vi "Part 2.vi"(11 "Input":string) -> (3 "Output":i64)   [LabVIEW 2021]
uses:
  b049b533-3b1e-4f4f-af40-132109b76cf6.vi
  <userlib>/_OpenG.lib/string/string.llb/Convert EOLs (String)__ogtk.vi
panel:
  in  "Numeric":i32=20
  out "Rocks":i32
  out "XY Graph":cluster{i32[], i32[]}[](graph)
  out "Time":dbl
  out "Pass?":bool
  in  "Test":i32
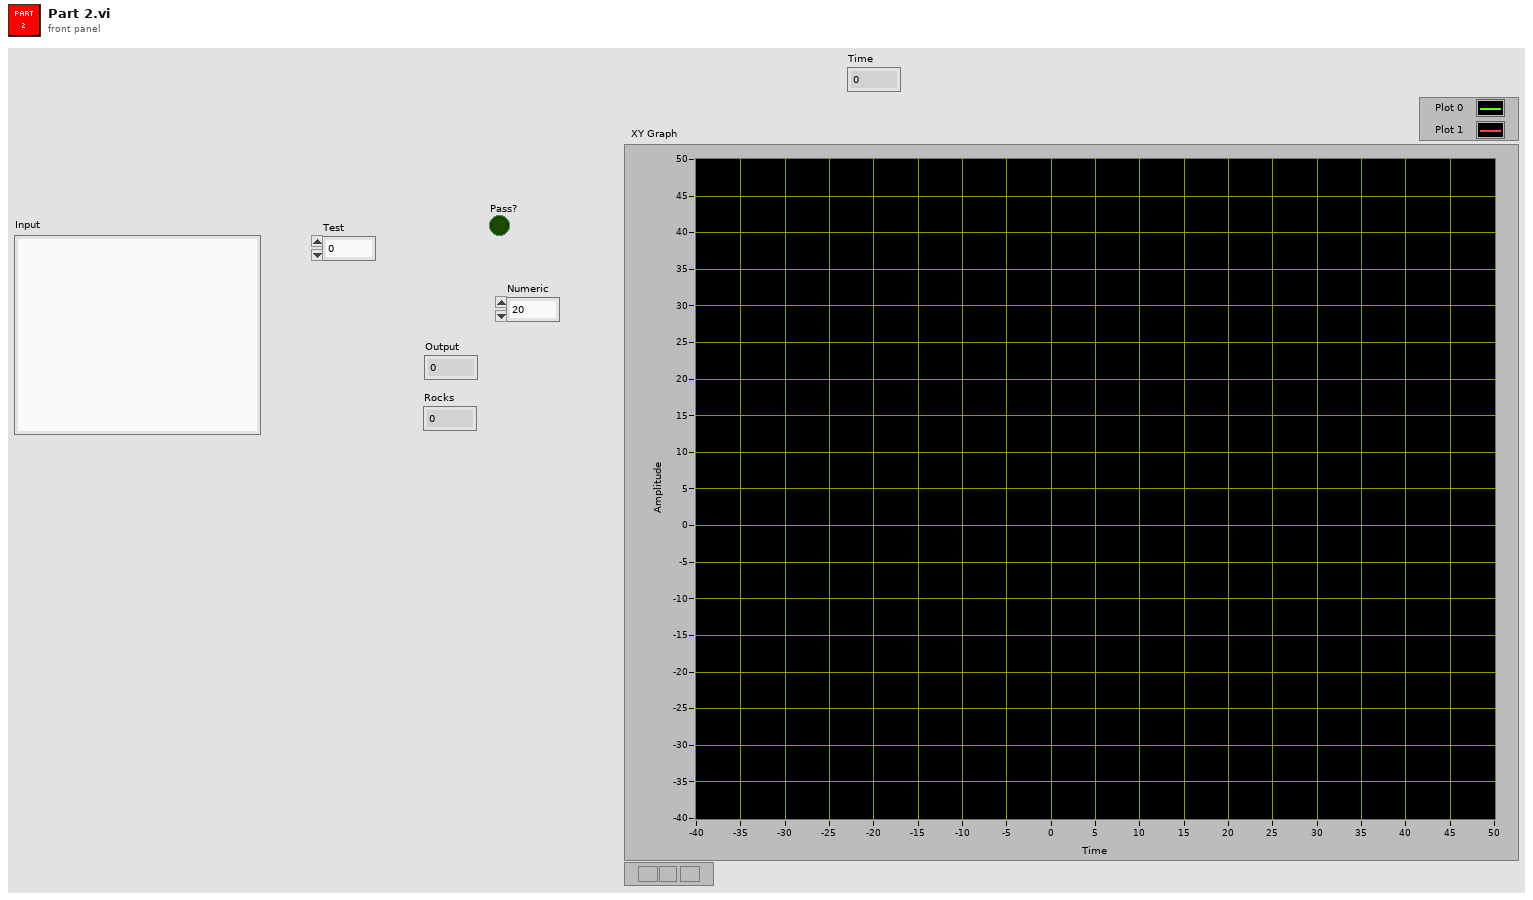
[diagram p1: front panel]
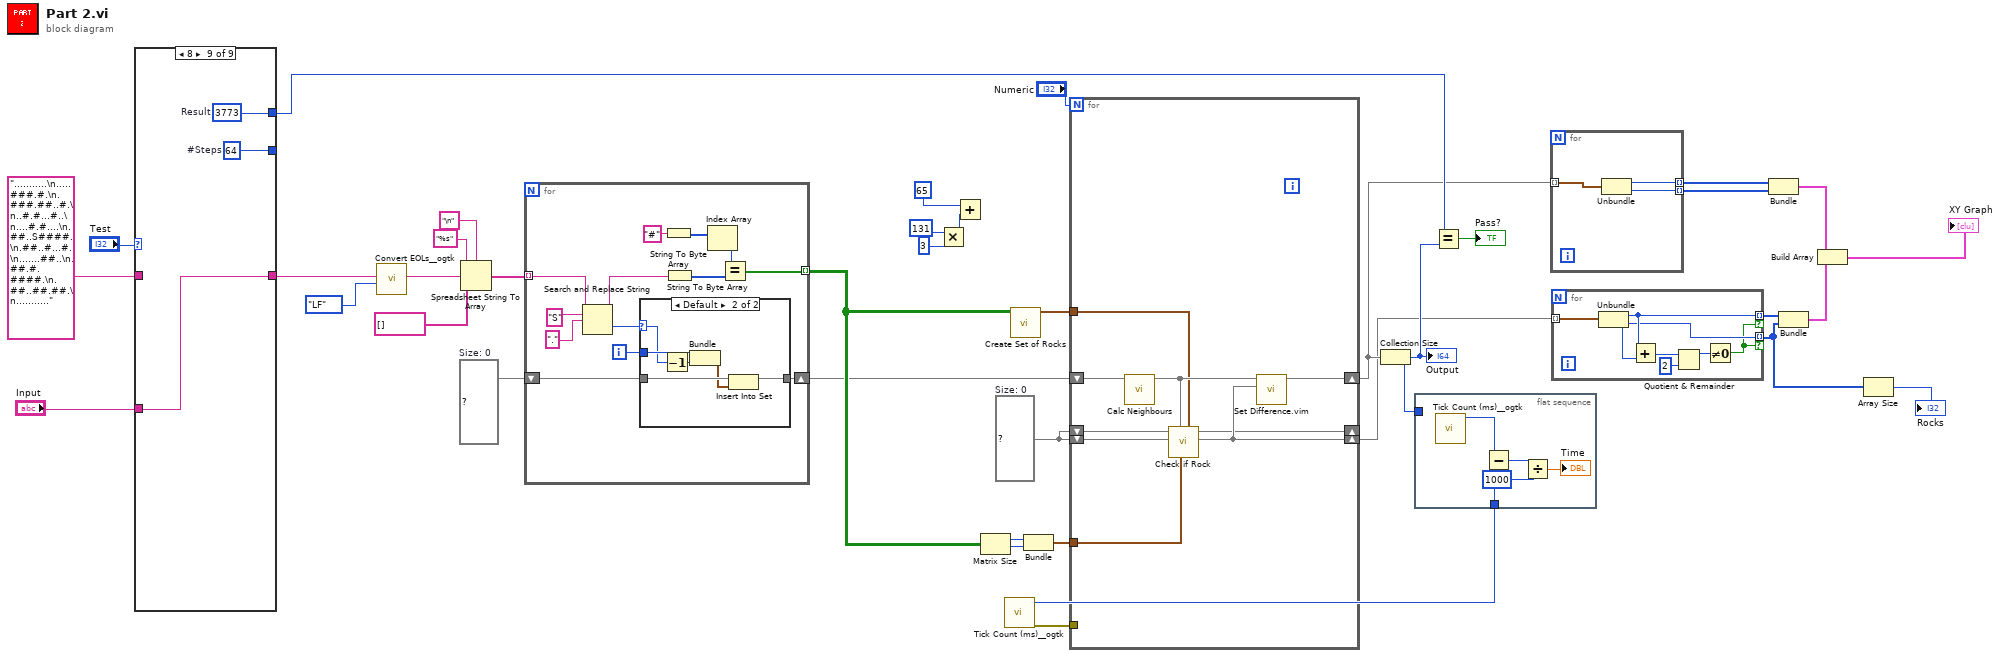
[diagram p0: block diagram]
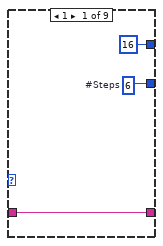
[diagram p2: hidden frame]
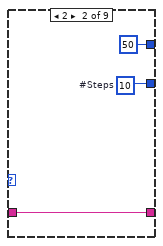
[diagram p3: hidden frame]
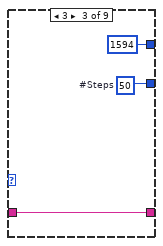
[diagram p4: hidden frame]
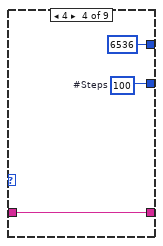
[diagram p5: hidden frame]
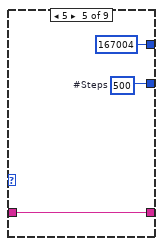
[diagram p6: hidden frame]
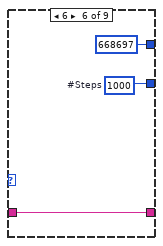
[diagram p7: hidden frame]
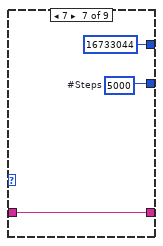
[diagram p8: hidden frame]
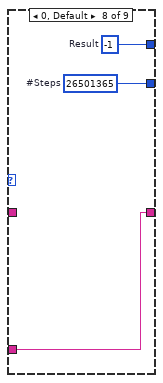
[diagram p9: hidden frame]
diagram:
  w16 = set{cluster{i32, i32}} {}  # Size: 0
  w18 = set{cluster{i32, i32}} {}  # Size: 0
  n1 = case shown="8" "Test" {
    tunnel: [w41 w44 w47 w50 w53 w56 w59 w60 w63] -> w38
    tunnel: [w40 w43 w46 w49 w52 w55 w58 w62 w65] -> _
    tunnel: "...........\n.....###.#.\n.###.##..#.\n..#.#...#..\n....#.#....\n.##..S####.\n.##..#...#.\n.......##..\n.##.#.####.\n.##..##.##.\n..........." -> [w41 w44 w47 w50 w53 w56 w59 _ _]
    tunnel: [16 ("Result") 50 ("Result") 1594 ("Result") 6536 ("Result") 167004 ("Result") 668697 ("Result") 16733044 ("Result") w61 w64] -> w28
    tunnel: "Input" -> [_ _ _ _ _ _ _ w60 w63]
    frame 1 {
      w40 = 6  # #Steps
    }
    frame 2 {
      w43 = 10  # #Steps
    }
    frame 3 {
      w46 = 50  # #Steps
    }
    frame 4 {
      w49 = 100  # #Steps
    }
    frame 5 {
      w52 = 500  # #Steps
    }
    frame 6 {
      w55 = 1000  # #Steps
    }
    frame 7 {
      w58 = 5000  # #Steps
    }
    frame 0, Default {
      w61 = -1  # Result
      w62 = 26501365  # #Steps
    }
    frame 8 {
      w64 = 3773  # Result
      w65 = 64  # #Steps
    }
  }
  n2 = call-poly <userlib>:"Convert EOLs__ogtk.vi"("Convert to:"=enum16{"CR", "LF", "CRLF"}."LF", "String in"=w38) -> ("String out"=w34:string)  [unwired: 9 in]
  n3 = Spreadsheet String To Array(delimiter (Tab)="\n", format string="%s", spreadsheet string=w34, array type (2D Dbl)=string[] []) -> (array=w32:string[])
  n4 = for {
    tunnel: w32 -> [w72] mode=indexing
    tunnel: [w74] -> w26 mode=indexing
    shift-right: [w67] -> w17
    shift-left: w16 -> [w66]
    i -> [w68]
    n5 = Search and Replace String(input string=w72, search string="S", replace string=".") -> (result string=w73:string, offset past replacement=w69:i32)  [unwired: 5 in, 2 out]
    n6 = case shown="Default" w69 {
      selector: w69 -> [_ w84]
      tunnel: w68 -> [_ w85]
      tunnel: [w79 w82] -> w67
      tunnel: w66 -> [w79 w81]
      frame -1 {
      }
      frame Default {
        n7 = Decrement(x=w84) -> (x-1=w83:i32)
        n8 = Bundle(w85, w83) -> (w80:cluster{i32, i32})  [unwired: 1 in]
        n9 = Insert Into Set(10:w80, 11:w81) -> (3:w82:set{cluster{i32, i32}})  [unwired: 1 out]
      }
    }
    n10 = String To Byte Array(string="#") -> (unsigned byte array=w77:u8[])
    n11 = String To Byte Array(string=w73) -> (unsigned byte array=w75:u8[])
    n12 = Index Array(array=w77) -> (element=w76:u8)  [unwired: 1 in]
    n13 = Equal?(x=w76, y=w75) -> (x = y?=w74:bool[])
  }
  n14 = Multiply(x=131, y=3) -> (x*y=w4:i32)
  n15 = Add(x=65, y=w4) -> ()  [unwired: 1 out]
  n16 = Matrix Size(0:w26) -> (1:w25:i32, 2:w24:i32)
  n17 = call <userlib>:"Tick Count (ms)__ogtk.vi"() -> ("error out"=w22:errorcluster, "millisecond timer value"=w20:u32)  [unwired: 10 in]
  n18 = call "Create Set of Rocks.vi"("Grid In"=w26) -> ("Rock Positions"=w27:cluster{i32, i32}[])  [unwired: 10 in]
  n19 = Bundle("number of columns"=w25, "matrix"=w24) -> (w23:cluster{"number of columns":i32, "matrix":i32})  [unwired: 1 in]
  n20 = for {
    N: "Numeric" -> [_]
    shift-right: [w86] -> w15
    shift-left: w17 -> [w94]
    tunnel: w27 -> [w90]
    tunnel: w23 -> [w89]
    shift-right: [w93] -> w9
    shift-left: w18 -> [w87]
    tunnel: w22 -> [_]
    shift-right: [w92] -> _
    shift-left: w18 -> [w88]
    n21 = call "Calc Neighbours.vi"("Set in"=w94) -> ("Set out"=w91:set{cluster{i32, i32}})  [unwired: 10 in]
    n22 = call "Check if Rock.vi"("Rock Positions"=w90, "Grid Size"=w89, "Current Positions"=w91, "Knowns Rocks"=w87, "Known Good Positions In"=w88) -> ("Known Rocks Out"=w93:set{cluster{i32, i32}}, "Known Good Positions Out"=w92:set{cluster{i32, i32}})  [unwired: 5 in]
    n23 = call "Set Difference.vim"("set 2"=w93, "set 1"=w91) -> ("difference"=w86:set{cluster{i32, i32}})  [unwired: 9 in]
  }
  n24 = Collection Size(1:w15) -> (0:w21:i32)
  "Output" <- w21
  n25 = flat-sequence {
    tunnel: w21 -> [_]
    tunnel: w20 -> [w98]
    frame #0 {
      n26 = call <userlib>:"Tick Count (ms)__ogtk.vi"() -> ("millisecond timer value"=w99:u32)  [unwired: 10 in, 1 out]
      n27 = Subtract(x=w99, y=w98) -> (x-y=w97:u32)
      n28 = Divide(x=w97, y=u32 1000) -> (x/y=→"Time":dbl)
    }
  }
  n29 = Equal?(x=w28, y=w21) -> (x = y?=→"Pass?":bool)
  n30 = for {
    tunnel: w15 -> [w102] mode=indexing
    tunnel: [w101] -> w14 mode=indexing
    tunnel: [w100] -> w13 mode=indexing
    n31 = Unbundle(w102) -> (w101:i32, w100:i32)
  }
  n32 = for {
    tunnel: w9 -> [w109] mode=indexing
    tunnel: [w108] -> w12 mode=indexing if=w103
    tunnel: [w107] -> w6 mode=indexing if=w103
    n33 = Unbundle(w109) -> (w108:i32, w107:i32)
    n34 = Add(x=w108, y=w107) -> (x+y=w106:i32)
    n35 = Quotient & Remainder(x=w106, y=2) -> (x-y*floor(x/y)=w104:i32)  [unwired: 1 out]
    n36 = Not Equal To 0?(x=w104) -> (x != 0?=w103:bool)
  }
  n37 = Bundle(w14, w13) -> (w11:cluster{i32[], i32[]})  [unwired: 1 in]
  n38 = Bundle(w12, w6) -> (w8:cluster{i32[], i32[]})  [unwired: 1 in]
  n39 = Build Array(w11, w8) -> (→"XY Graph":cluster{i32[], i32[]}[])
  n40 = Array Size(array=w6) -> (size(s)=→"Rocks":i32)
